vi "WriteerrorLog.vi"() -> ()   [LabVIEW 2024]
panel:
  out "Valid File?":bool
  out "Error_Log":path
  in  "Error String":string
  out "error out":errorcluster
  in  "error in":errorcluster
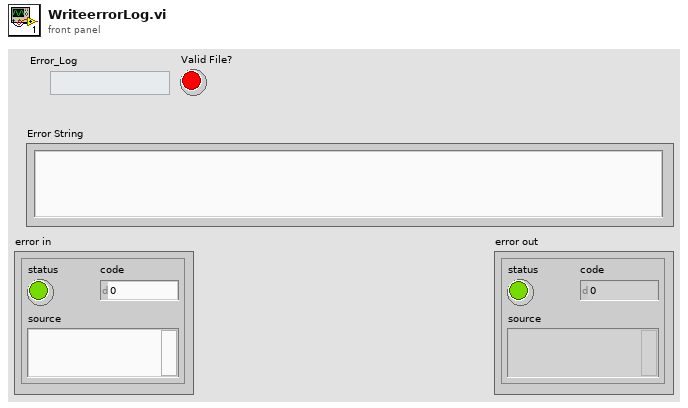
[diagram p1: front panel]
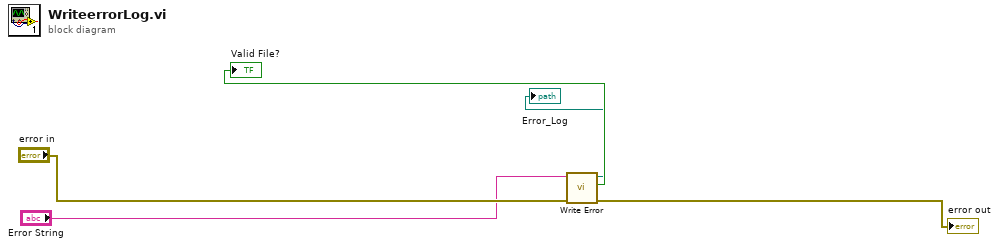
[diagram p0: block diagram]
diagram:
  n1 = call "Write Error.vi"("error in (no error)"="error in", "Error String"="Error String") -> ("error out"=→"error out":errorcluster, "Valid File?"=→"Valid File?":bool, "Error_Log"=→"Error_Log":path)  [unwired: 7 in]
